vi "paste_kinematic_data.vi"() -> ()   [LabVIEW 2014]
uses:
  testing/manipulator_cal.ctl
  asap/labview/testing/probe_calibration.ctl
  initialization/micron_globals.vi
panel:
  out "Result":dbl[][][](array[numeric])
  out "Manipulator calibration":T1={"Tool offsets"=[[0.0, 0.0, 36200.0]], "Handle light calibration"=[], "Base pivots"=[], "Output pivots"=[], "Length center"=0.0, "Workspace height"=[0.0, 0.0, 36200.0], "Workspace diameter"=[0.0, 0.0, 36200.0], "Stack travel"=400.0, "Saturation pos"=375.0, "Inverse filters"=[], "Strut length"=0.0, "Tip light calibration"=[]} {"Tip light calibration" format="%#.1f"; "Strut length" format="%#_4p"; "Saturation pos" format="%#.1f"; "Stack travel" format="%#.1f"; "Length center" format="%#_4p"; "Output pivots" format="%#_6f"; "Base pivots" format="%#_6f"; "Handle light calibration" format="%#.1f"}
  # "This VI is used to initialize the manipulator kinematic data,\ntypically from data copied from excel.  Paste this into the string\nconstants on the block diagram and run this, then save\nthe config."
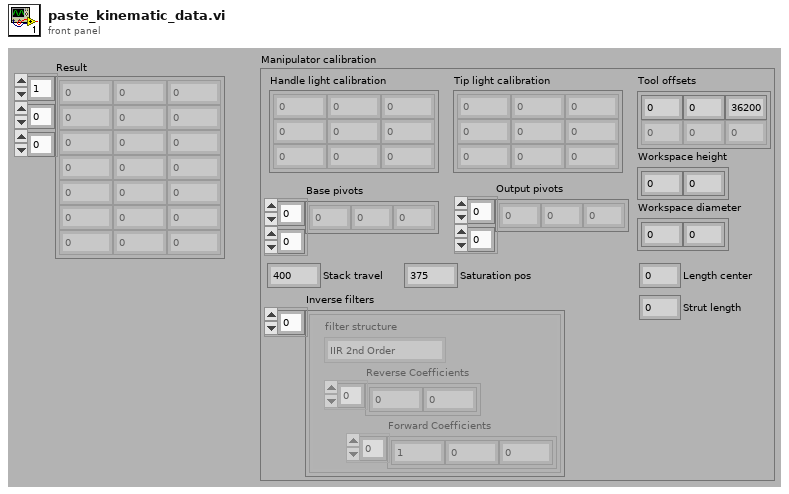
[diagram p1: front panel]
types:
  T1 = typedef "manipulator_cal.ctl" = cluster{"Tool offsets":sgl[][], "Handle light calibration":T2, "Base pivots":sgl[][], "Output pivots":sgl[][], "Length center":sgl, "Workspace height":sgl[], "Workspace diameter":sgl[], "Stack travel":sgl, "Saturation pos":sgl, "Inverse filters":cluster{"filter structure":enum32{"IIR 2nd Order", "IIR 4th Order"}, "Reverse Coefficients":dbl[], "Forward Coefficients":dbl[]}[], "Strut length":sgl, "Tip light calibration":T2}
  T2 = typedef "probe_calibration.ctl" = sgl[][]
  T3 = typedef "Micron params.ctl" = cluster{"Stimulus":T4, "Goal Filter A":T6, "Mode controls":T7, "Manipulator type":enum16{"Current piezo", "Voltage piezo"}, "Manipulator calibration":T1, "Network":T8, "Goal Filter B":T6, "Cancellation":T9, "Transition time":sgl, "Estimation":T11}
  T4 = typedef "stimulus.ctl" = cluster{"Type":enum16{"Off", "Step", "Sine", "Triangle", "Arbitrary"}, "Phase":dbl, "Amplitude":sgl[], "Injection point":T5, "Closed loop":bool, "Offset":sgl[], "Tip -> world":bool, "Frequency":dbl, "Length":dbl}
  T5 = typedef "injection_point.ctl" = enum16{"Total pose", "V limiter", "Goal ", "Link position", "KF link position", "Inverse kin", "Link goal", "Link error", "Controller", "Output", "Drive", "Light"}
  T6 = typedef "goal_loop_parms.ctl" = cluster{"Speedup max":sgl, "Speedup thresh":sgl, "Speedup nonlin":sgl, "Filters":cluster{"Lower Fc":sgl, "Lower Q":sgl, "Scale factor":sgl, "Upper Fc":sgl, "Upper Q":sgl, "V limit":sgl, "V limit range":sgl}[]}
  T7 = typedef "mode_conrols.ctl" = cluster{"Hold":bool, "Cancellation":bool, "Goal filter":bool, "Trigger":bool}
  T8 = typedef "network_params.ctl" = cluster{"Remote Host":string, "Send Status":bool, "Send Port":u16, "Recv Commands":bool, "Recv Port":u16}
  T9 = typedef "sq_control_params.ctl" = cluster{"KP":T10, "KI":sgl, "KD":T10, "Max vel":sgl, "Max acc":sgl, "Int error limit":sgl, "RCM gain":sgl, "Bypass":bool, "Degraded gain":sgl}
  T10 = typedef "decoupled_gain.ctl" = cluster{"XY":sgl, "Rxy":sgl, "Z":sgl, "Rz":sgl}
  T11 = typedef "estimation_controls.ctl" = cluster{"Link":cluster{"Measure noise":dbl[], "Process noise":dbl[], "Alt process noise":dbl[], "Alt turnoff cycles":i32, "Innovation limit":dbl[], "Residue threshold":dbl, "Enable":bool}, "Handle":cluster{"Measure noise":dbl[], "Process noise":dbl[], "State limits":dbl[], "Innovation limit":dbl[], "Prediction Lookahead":sgl, "Enable":bool}}
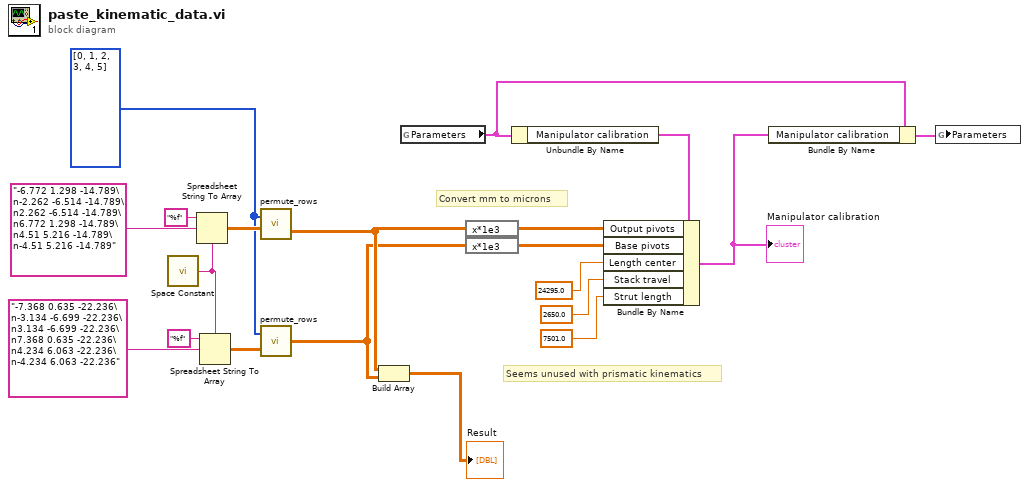
[diagram p0: block diagram]
diagram:
  w9 = i32[] [0, 1, 2, 3, 4, 5] ("x-y")
  # "Seems unused with prismatic kinematics"
  # "Convert mm to microns"
  n1 = call <vilib>:"Space Constant.vi"() -> ("String"=w5:string)
  n2 = Spreadsheet String To Array(delimiter (Tab)=w5, format string="%f", spreadsheet string="-6.772 1.298 -14.789\n-2.262 -6.514 -14.789\n2.262 -6.514 -14.789\n6.772 1.298 -14.789\n4.51 5.216 -14.789\n-4.51 5.216 -14.789") -> (array=w11:dbl[][])  [unwired: 1 in]
  n3 = Spreadsheet String To Array(delimiter (Tab)=w5, format string="%f", spreadsheet string="-7.368 0.635 -22.236\n-3.134 -6.699 -22.236\n3.134 -6.699 -22.236\n7.368 0.635 -22.236\n4.234 6.063 -22.236\n-4.234 6.063 -22.236") -> (array=w10:dbl[][])  [unwired: 1 in]
  n4 = call "permute_rows.vi"("Array"=w11, "Permutation"=w9) -> ("Result"=w3:dbl[][])
  n5 = call "permute_rows.vi"("Array"=w10, "Permutation"=w9) -> ("Result"=w2:dbl[][])
  n6 = Build Array(w3, w2) -> (→"Result":dbl[][][])
  n7 = global read "micron_globals.vi" "Parameters"() -> (w15:T3)
  n8 = expression code="x*1e3"(w3) -> (w12:dbl[][])
  n9 = expression code="x*1e3"(w2) -> (w13:dbl[][])
  n10 = Unbundle By Name(w15) -> ("Manipulator calibration"=w16:T1)
  n11 = Bundle By Name(cluster=w16, "Output pivots"=w12, "Base pivots"=w13, "Length center"=24295.0 ("magnitude"), "Stack travel"=sgl 2650.0, "Strut length"=sgl 7501.0 ("Saturation pos")) -> (w6:T1)
  "Manipulator calibration" <- w6
  n12 = Bundle By Name(cluster=w15, "Manipulator calibration"=w6) -> (w14:T3)
  n13 = global write "micron_globals.vi" "Parameters"(w14) -> ()
